vi "Test FlexiFlowInterfaceCH2 API.vi"() -> ()   [LabVIEW 2025]
doc: "FlexiFlowInterfaceCH2 API Tester."
uses:
  <vilib>/MGI/Panel Manager/Panel/Panel.lvlib
  <vilib>/MGI/Panel Manager/Panel/Panel/Window/Window.vi
  <vilib>/MGI/Panel Manager/Panel/Panel/Window/Window.lvclass
  <vilib>/MGI/Panel Manager/Panel/Panel/Subpanel/Subpanel.vi
  <vilib>/MGI/Panel Manager/Panel/Panel/Subpanel/Subpanel.lvclass
  <vilib>/MGI/Panel Manager/Panel/Panel/Window/Dialog/Dialog.vi
  <vilib>/MGI/Panel Manager/Panel/Panel/Window/Dialog/Dialog.lvclass
  C:/Program Files/National Instruments/LabVIEW 2025/vi.lib/MGI/Panel Manager/Panel/Panel/Panel.lvclass
  C:/Program Files/National Instruments/LabVIEW 2025/vi.lib/MGI/Panel Manager/Panel/Panel/Window/Window.lvclass
  C:/Program Files/National Instruments/LabVIEW 2025/vi.lib/MGI/Panel Manager/Panel/Panel/Window/Dialog/Dialog.lvclass
  C:/Program Files/National Instruments/LabVIEW 2025/vi.lib/MGI/Panel Manager/Panel/Panel/Subpanel/Subpanel.lvclass
  FlexiFlowInterface/Modbus TCP Connection Settings--cluster.ctl
  FlexiFlowInterface/FlexiFlowDevice--enum.ctl
  phlair-shared-libraries/Modbus Flexi-Flow API/Control Function Values--enum.ctl
  phlair-shared-libraries/Modbus Flexi-Flow API/Bronkhorst Flexi-Flow ModbusTCP API.lvlib
  FlexiFlowInterface/Modbus Flexi-Flow Controls--cluster.ctl
  FlexiFlowInterface/Modbus Flexi-Flow Measure State--cluster.ctl
  <vilib>/Plasmionique/MB Master/MB_Master_TCP/MB_Master_TCP.lvclass
  FlexiFlowInterface/Modbus Flexi-Flow State--cluster.ctl
  phlair-shared-libraries/Modbus Flexi-Flow API/Counter Setpoint Mode--enum.ctl
  phlair-shared-libraries/Modbus Flexi-Flow API/Counter Modes--enum.ctl
  FlexiFlowInterface/Counter Settings--cluster.ctl
  phlair-shared-libraries/Modbus Flexi-Flow API/Control Mode--enum.ctl
  phlair-shared-libraries/Modbus Flexi-Flow API/Capacity Units (Standard Volume Flow).ctl
  FlexiFlowInterface/Device Type--enum.ctl
panel:
  in  "Tab Control":T1(tab)
  out "Module Running?":bool
  in  "Show Module Panel":bool
  in  "Hide Module Panel":bool
  in  "Start Module":bool
  in  "Stop Module":bool
  in  "Show Block Diagram":bool
  in  "Tab Control":enum32{"Status", "Subpanel"}(tab)
  out "Status":string
  in  "Autoshow?":bool
  in  "Panel Type":enum16{"Window", "Dialog", "Subpanel"}(ring)
  in  "Change Panel":bool
  in  "Initialise Modbus Connections":bool
  in  "Wink Devices":bool
  in  "Flexi-Flow Conn":T2[](array[typedef])=[{"Label"="H2_PR", "Slave ID (255)"=255, "IP Address"="192.168.100.10", "Port (502)"=502, "Timeout (10000)"=2000}, {"Label"="N2_PR", "Slave ID (255)"=255, "IP Address"="192.168.100.20", "Port (502)"=502, "Timeout (10000)"=2000}, {"Label"="C_MFM", "Slave ID (255)"=255, "IP Address"="192.168.100.30", "Port (502)"=502, "Timeout (10000)"=2000}, {"Label"="A_MFC", "Slave ID (255)"=255, "IP Address"="192.168.100.40", "Port (502)"=502, "Timeout (10000)"=2000}]
  in  "Setpoint Slope":u16
  in  "Set Setpoint Slope":bool
  in  "Set Flow Capacity Unit":bool
  in  "Forwardpressure SP":dbl
  in  "Set Forward Pressure SP":bool
  in  "Backpressure SP":dbl
  in  "Set Backpressure Setpoint":bool
  in  "Flow SP":dbl
  in  "Set Flow SP":bool
  in  "Function":T3=enum."Downstream pressure"
  in  "Set Control Function":bool
  in  "Control Mode":T4 items=["Bus/RS232"=0, "FLOW-BUS slave"=2, "Valve close"=3, "Controller idle"=4, "Setpoint 100%"=7, "Valve fully open"=8, "Calibration mode"=9, "Setpoint 0%"=12, "RS232"=18, "Valve steering"=20, "Valve safe state"=22]
  in  "Set Control Mode":bool
  in  "User Tag":string
  in  "Set Device User Tag":bool
  in  "Device":T5
  in  "Standard Volume Flow":T6=4 items=["uls/h", "uls/min", "uls/s", "mls/h", "mls/min", "mls/s", "ls/h", "ls/min", "ls/s", "ccs/h", "ccn/min", "ccs/s", "mm3s/h", "mm3s/m", "mm3s/s", "cm3s/h", "cm3s/m", "cm3s/s", "m3s/h", "m3s/min", "m3s/s"]
  in  "Get Device Configuration":bool
  in  "Read Counter Unit":bool
  in  "Read Device User Tag":bool
  in  "Wink Device":bool
  in  "Read Fmeasure":bool
  out "Flexi-Flow Devices":T7[](array[typedef]) {"Control State"."Control Mode" items=["Bus/RS232"=0, "FLOW-BUS slave"=2, "Valve close"=3, "Controller idle"=4, "Setpoint 100%"=7, "Valve fully open"=8, "Calibration mode"=9, "Setpoint 0%"=12, "RS232"=18, "Valve steering"=20, "Valve safe state"=22]}
  in  "Device 2":T5 caption="Device"
  out "Data Table":map{string, dbl}(c390)
  in  "Counter Settings":T11={"Counter Setpoint Mode"=enum."No setpoint change (default)", "Counter Limit"=0.0, "Unit"="ls", "Counter Mode"=enum."Counter off (default)", "Counter New Setpoint"=0}
  in  "Reset All Device Counters":bool
  in  "Set Counter Settings":bool
  in  "Modbus TCP Connection":T2={"Label"="", "Slave ID (255)"=255, "IP Address"="192.168.100.10", "Port (502)"=502, "Timeout (10000)"=10000}
  in  "Set Modbus Configuration":bool
  # "This VI tests the API for the Module."
  # "Change Panel"
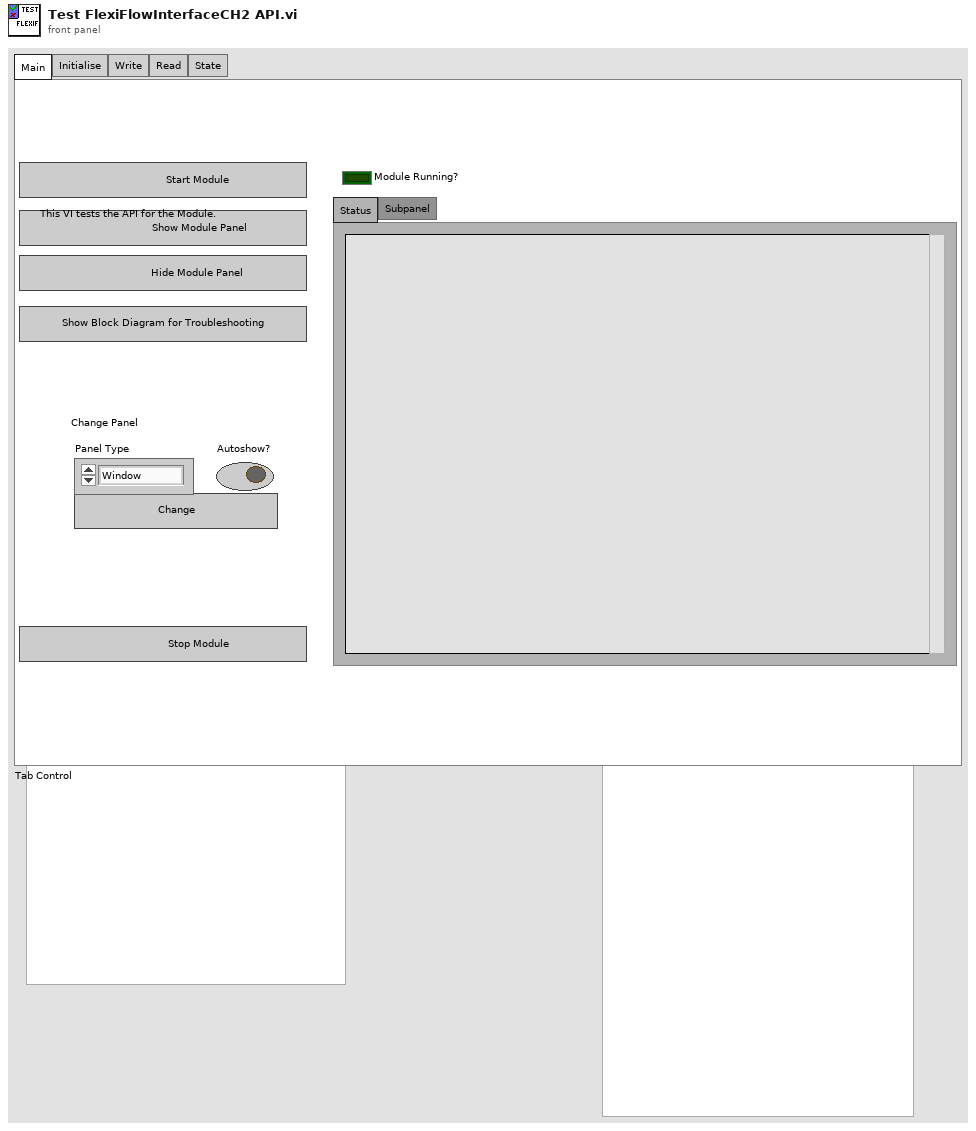
[diagram p1: front panel]
types:
  T1 = enum32{"Main", "Initialise", "Write", "Read", "State"}
  T2 = typedef "FlexiFlowInterface.lvlib/Modbus TCP Connection Settings--cluster.ctl" = cluster{"Label":string, "Slave ID (255)":u8, "IP Address":string, "Port (502)":u16, "Timeout (10000)":i32}
  T3 = typedef "Bronkhorst Flexi-Flow ModbusTCP API.lvlib/Control Function Values--enum.ctl" = enum16{"Flow", "Upstream pressure", "Downstream pressure", "Flow with upstream pressure limit", "Flow with downstream pressure limit", "Upstream pressure with flow limit", "Downstream pressure with flow limit"}
  T4 = typedef "Bronkhorst Flexi-Flow ModbusTCP API.lvlib/Control Mode--enum.ctl" = u16
  T5 = typedef "FlexiFlowInterface.lvlib/FlexiFlowDevice--enum.ctl" = enum16{"Hydrogen Inlet", "Nitrogen Inlet", "Cathode Outlet", "Anode Outlet"}
  T6 = typedef "Bronkhorst Flexi-Flow ModbusTCP API.lvlib/Capacity Units (Standard Volume Flow).ctl" = u16
  T7 = typedef "FlexiFlowInterface.lvlib/Modbus Flexi-Flow State--cluster.ctl" = cluster{"Type":T8, "Label":string, "User Tag":string, "MB_TCP session":refnum<class "MB_Master_TCP.lvclass">, "Control State":T9, "Measurement State":T10}
  T8 = typedef "FlexiFlowInterface.lvlib/Device Type--enum.ctl" = enum16{"Mass Flow Controller", "Mass Flow Meter"}
  T9 = typedef "FlexiFlowInterface.lvlib/Modbus Flexi-Flow Controls--cluster.ctl" = cluster{"Control Mode":T4, "Function":T3, "FSetpoint":sgl, "Flow Capacity Unit":string, "Setpoint Slope":u16, "P1Setpoint":sgl, "P2Setpoint":sgl}
  T10 = typedef "FlexiFlowInterface.lvlib/Modbus Flexi-Flow Measure State--cluster.ctl" = cluster{"Fmeasure":dbl, "P1measure":sgl, "P2measure":sgl}
  T11 = typedef "FlexiFlowInterface.lvlib/Counter Settings--cluster.ctl" = cluster{"Counter Setpoint Mode":T12, "Counter Limit":sgl, "Unit":string, "Counter Mode":T13, "Counter New Setpoint":u16}
  T12 = typedef "Bronkhorst Flexi-Flow ModbusTCP API.lvlib/Counter Setpoint Mode--enum.ctl" = enum16{"No setpoint change (default)", "Change setpoint to Counter new setpoint"}
  T13 = typedef "Bronkhorst Flexi-Flow ModbusTCP API.lvlib/Counter Modes--enum.ctl" = enum16{"Counter off (default)", "Counting up continuously", "Counting up until limit reached"}
  T14 = typedef "FlexiFlowInterface.lvlib/Broadcast Events--cluster.ctl" = cluster{"Module Did Init":refnum<user-event>, "Status Updated":refnum<user-event>, "Error Reported":refnum<user-event>, "Module Did Stop":refnum<user-event>, "Update Module Execution Status":refnum<user-event>, "Broadcast Device States":refnum<user-event>, "Broadcast State (Data Map)":refnum<user-event>}
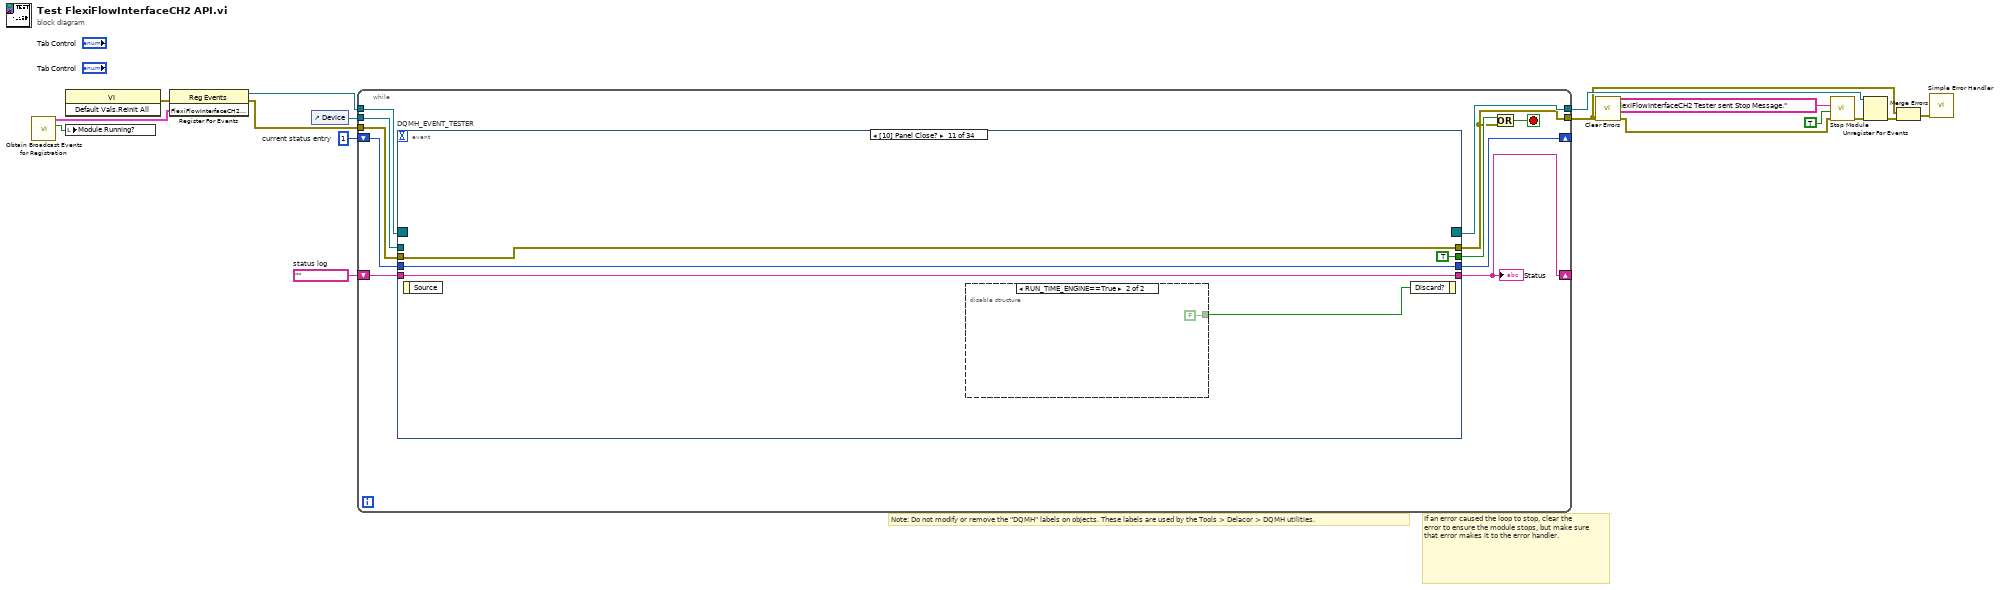
[diagram p0: block diagram]
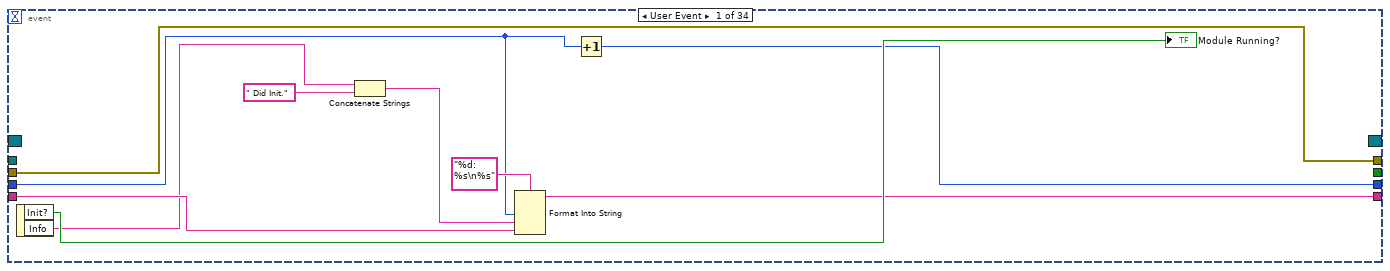
[diagram p2: hidden frame]
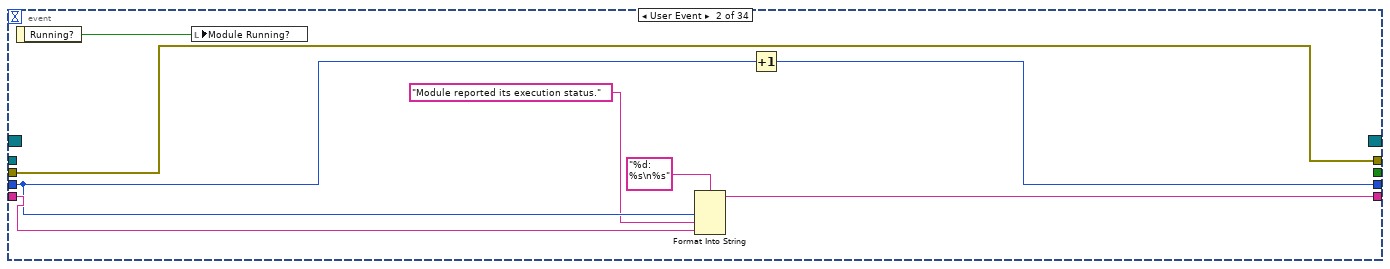
[diagram p3: hidden frame]
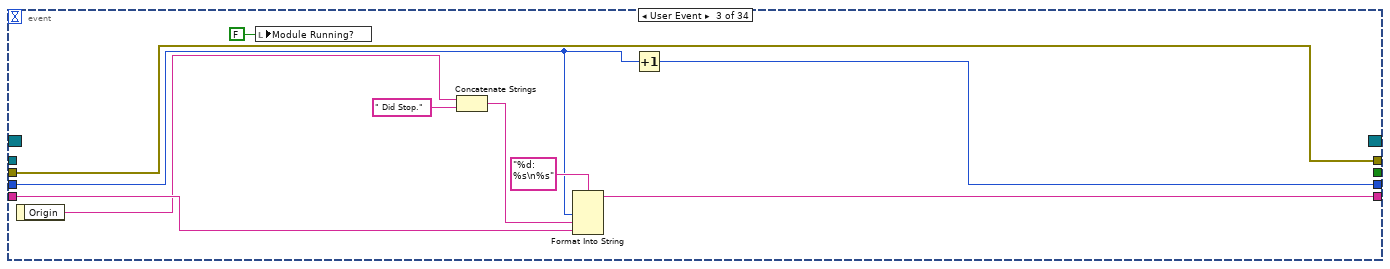
[diagram p4: hidden frame]
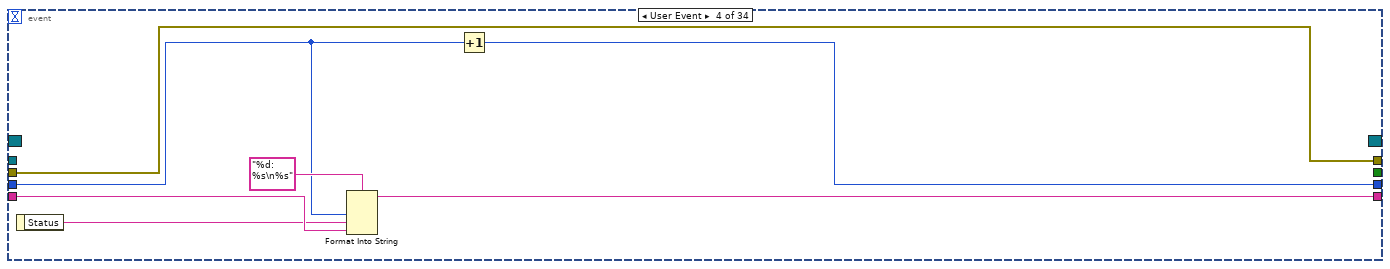
[diagram p5: hidden frame]
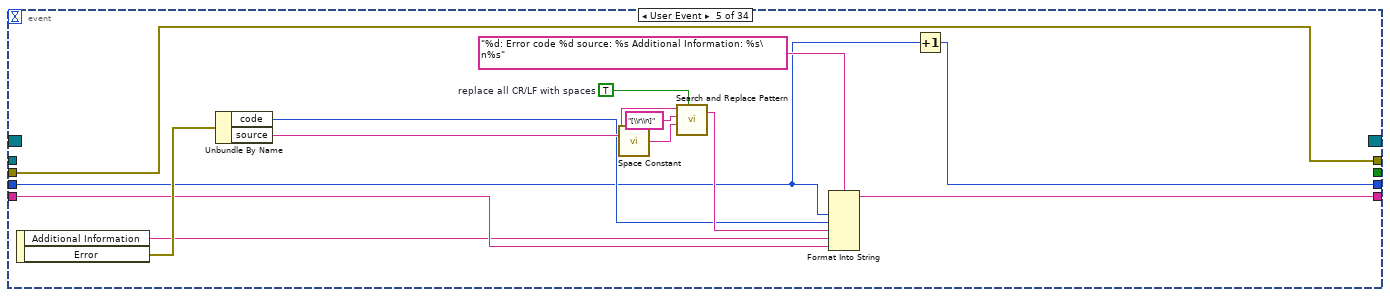
[diagram p6: hidden frame]
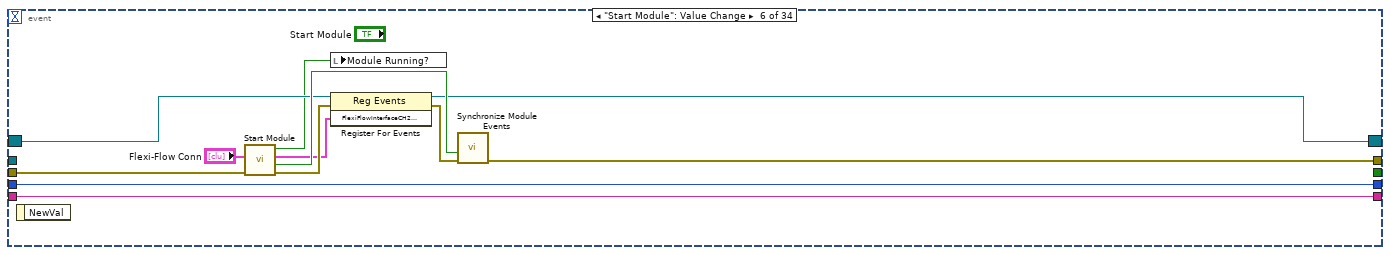
[diagram p7: hidden frame]
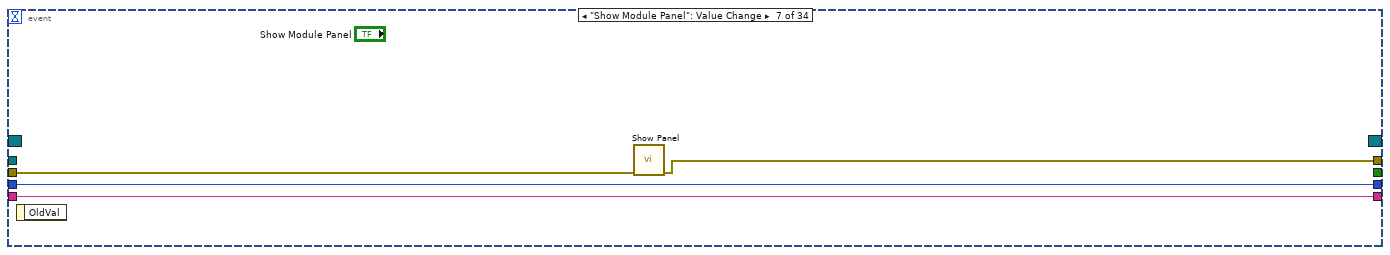
[diagram p8: hidden frame]
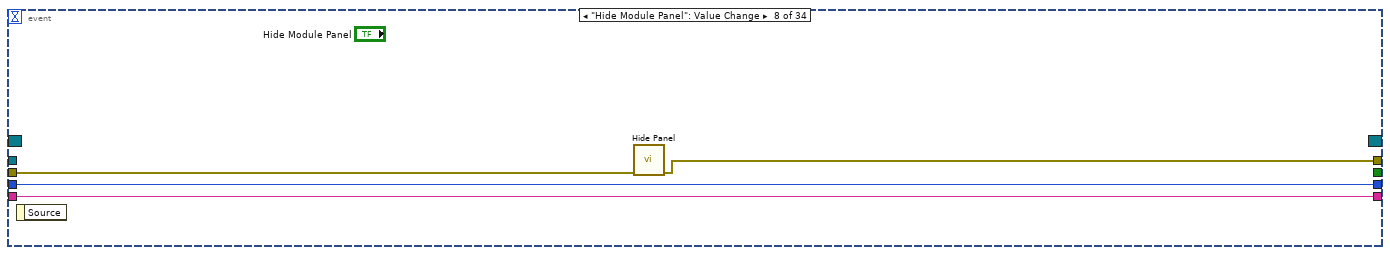
[diagram p9: hidden frame]
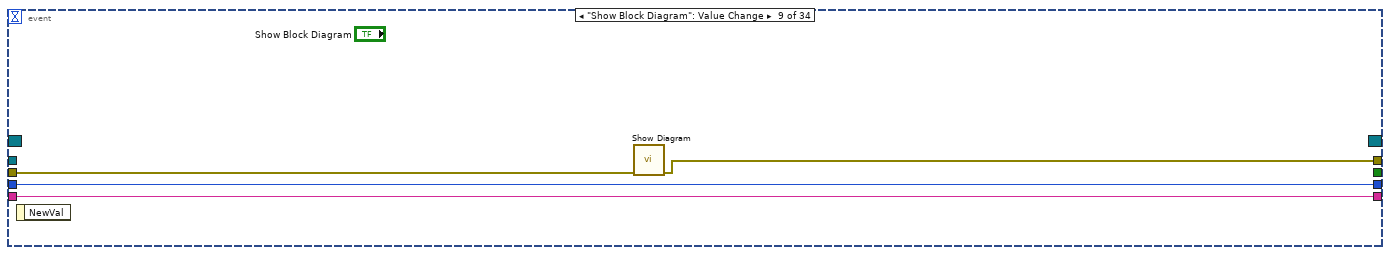
[diagram p10: hidden frame]
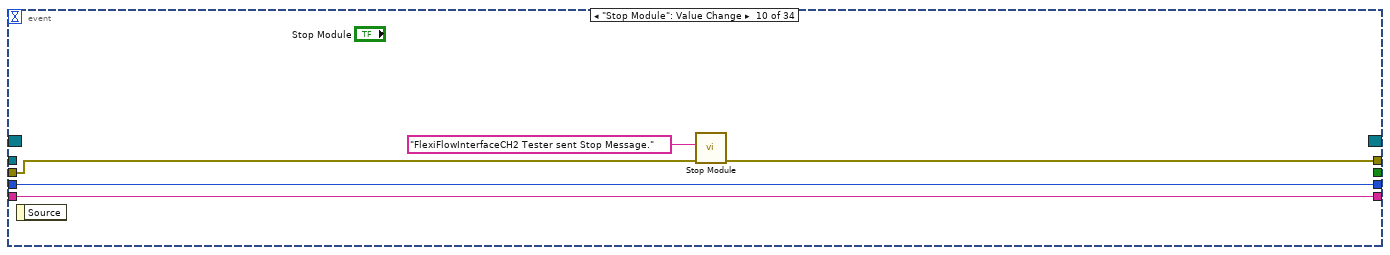
[diagram p11: hidden frame]
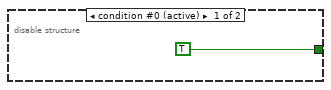
[diagram p12: hidden frame]
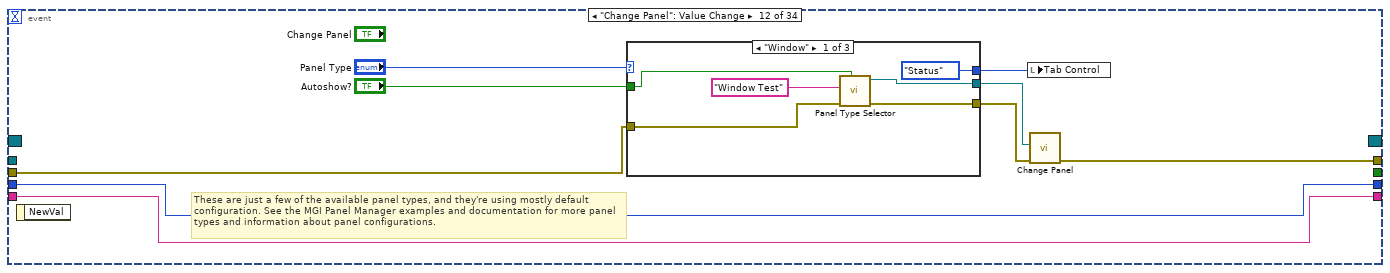
[diagram p13: hidden frame]
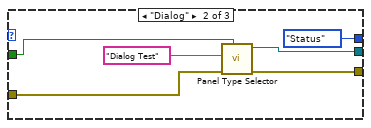
[diagram p14: hidden frame]
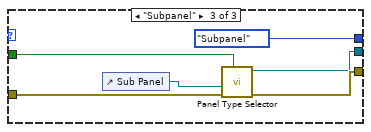
[diagram p15: hidden frame]
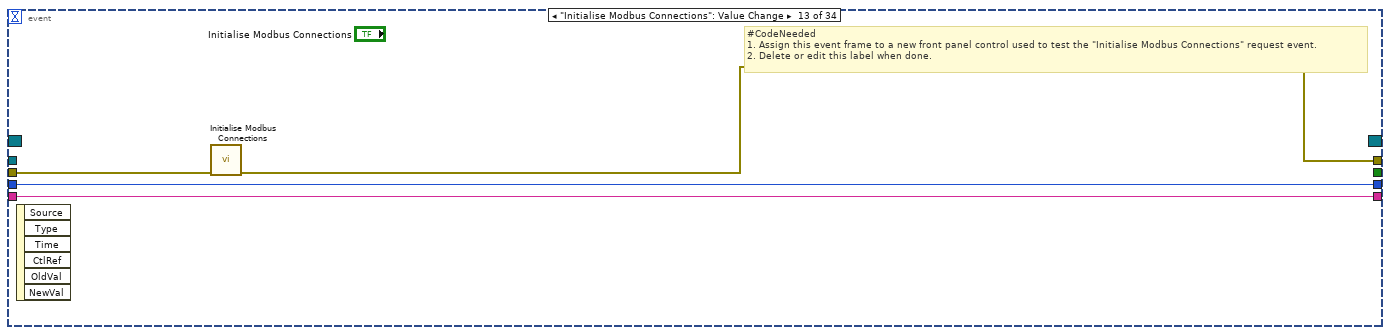
[diagram p16: hidden frame]
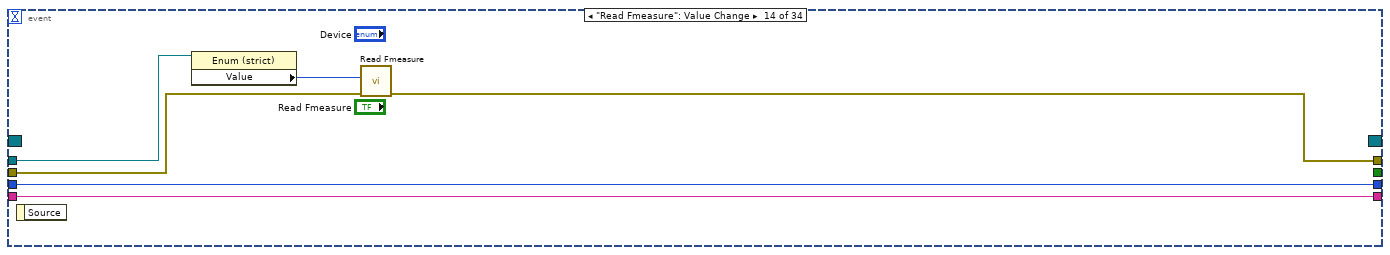
[diagram p17: hidden frame]
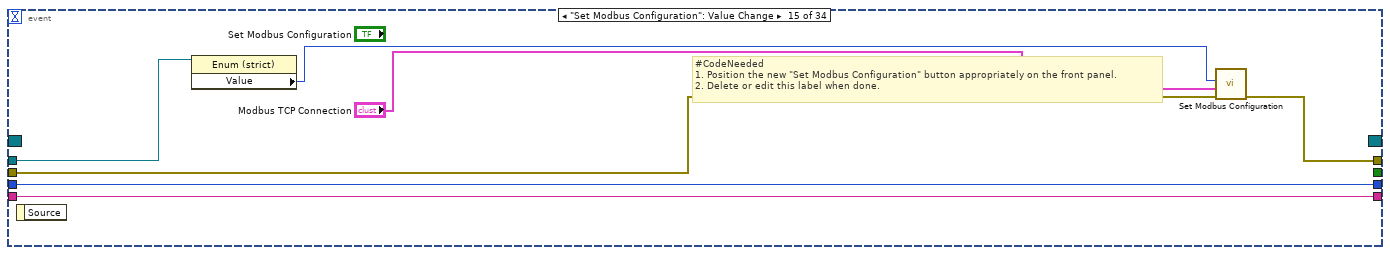
[diagram p18: hidden frame]
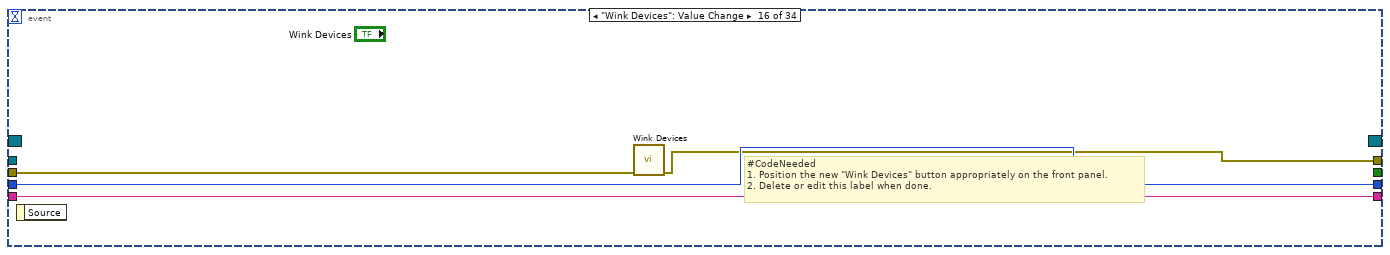
[diagram p19: hidden frame]
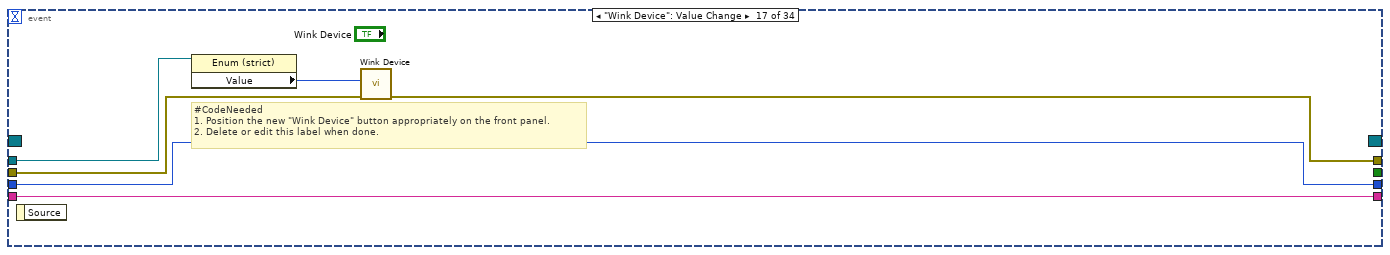
[diagram p20: hidden frame]
diagram:
  w12 = 1  # current status entry
  w13 = ""  # status log
  # "If an error caused the loop to stop, clear the error to ensure the module stops, but make sure that error makes it to the error handler."
  # "Note: Do not modify or remove the \"DQMH\" labels on objects. These labels are used by the Tools > Delacor > DQMH utilities."
  n1 = call "Obtain Broadcast Events for Registration.vi"() -> ("Already running?"=w2:bool, "FlexiFlowInterfaceCH2 Broadcast Events"=w9:T14)  [unwired: 9 in, 1 out]
  n2 = invoke class="VI" method="Default Vals.Reinit All"() -> (error out=w11:errorcluster)  [unwired: 3 in, 2 out]
  n3 = local write "Module Running?"(w2) -> ()
  n4 = register-events(error in=w11, w9) -> (reference out=w8:refnum<event-registration>, error out=w10:errorcluster)  [unwired: 1 in]
  n5 = control-ref of="Device"() -> (w1:refnum<vi>)
  n6 = while {
    tunnel: w8 -> [w27]
    tunnel: [w18] -> w3
    shift-right: [w22] -> _
    shift-left: w13 -> [w24]
    shift-right: [w23] -> _
    shift-left: w12 -> [w25]
    tunnel: w10 -> [w20]
    tunnel: [w19] -> w7
    tunnel: w1 -> [w17]
    stop <- w21 stop-if-true
    n7 = event "DQMH_EVENT_TESTER" shown="[10] Panel Close?" {
      selector: w27 -> [_ _ _ _ _ w82 _ _ _ _ _ _ _ _ _ _ _ _ _ _ _ _ _ _ _ _ _ _ _ _ _ _ _ _]
      dyn-events: [_ _ _ _ _ w81 _ _ _ _ _ _ _ _ _ _ _ _ _ _ _ _ _ _ _ _ _ _ _ _ _ _ _ _] -> w19
      timeout: _ -> [_ _ _ _ _ _ _ _ _ _ _ _ _ _ _ _ _ _ _ _ _ _ _ _ _ _ _ _ _ _ _ _ _ _]
      tunnel: [_ _ _ _ _ _ _ _ _ _ TRUE ("Discard?") _ _ _ _ _ _ _ _ _ _ _ _ _ _ _ _ _ _ _ _ _ _ _] -> w26
      tunnel: [w37 w39 w46 w56 w76 w80 w92 w96 w97 w103 w107 w119 w140 w146 w153 w157 w163 w170 w177 w184 w191 w198 w205 w218 w228 w232 w236 w242 w249 w255 w262 w268 w275 w279] -> w18
      tunnel: w25 -> [w33 w43 w53 w59 w66 w85 w90 w94 w98 w104 w108 w120 w141 w147 w154 w158 w164 w171 w178 w185 w192 w199 w206 w215 w225 w233 w237 w243 w250 w256 w263 w269 w273 w277]
      tunnel: w24 -> [w34 w44 w54 w58 w64 w86 w91 w95 w99 w105 w109 w121 w142 w148 w155 w159 w165 w172 w179 w186 w193 w200 w207 w217 w227 w234 w238 w244 w251 w257 w264 w270 w274 w278]
      tunnel: [w31 w41 w51 w60 w67 w86 w91 w95 w99 w105 w109 w121 w142 w148 w155 w159 w165 w172 w179 w186 w193 w200 w207 w216 w226 w234 w238 w244 w251 w257 w264 w270 w274 w278] -> w22
      tunnel: [w32 w42 w52 w62 w65 w85 w90 w94 w98 w104 w108 w120 w141 w147 w154 w158 w164 w171 w178 w185 w192 w199 w206 w214 w224 w233 w237 w243 w250 w256 w263 w269 w273 w277] -> w23
      tunnel: w20 -> [w37 w39 w46 w56 w76 w78 w89 w93 w100 w101 w107 w118 w143 w149 w156 w160 w166 w173 w180 w187 w194 w201 w208 w218 w228 w235 w239 w245 w252 w258 w265 w271 w275 w279]
      tunnel: w17 -> [_ _ _ _ _ _ _ _ _ _ _ _ _ w145 w152 _ w161 w168 w176 w182 w190 w197 w203 _ _ w231 _ w240 w248 w254 w261 w266 _ _]
      event User Event {
        n8 = event-data() -> ("Init?"=→"Module Running?":bool, "Info"=w30:string)  [unwired: 1 in]
        n9 = Concatenate Strings(w30, " Did Init.") -> (w29:string)
        n10 = Format Into String(format string="%d: %s\n%s", w33, w29, w34) -> (resulting string=w31:string)  [unwired: 2 in, 1 out]
        n11 = Increment(x=w33) -> (x+1=w32:i32)
      }
      event User Event {
        n12 = event-data() -> ("Running?"=w38:bool)  [unwired: 1 in]
        n13 = local write "Module Running?"(w38) -> ()
        n14 = Format Into String(format string="%d: %s\n%s", w43, "Module reported its execution status.", w44) -> (resulting string=w41:string)  [unwired: 2 in, 1 out]
        n15 = Increment(x=w43) -> (x+1=w42:i32)
      }
      event User Event {
        n16 = event-data() -> ("Origin"=w50:string)  [unwired: 1 in]
        n17 = local write "Module Running?"(FALSE ("Module Did Init?")) -> ()
        n18 = Concatenate Strings(w50, " Did Stop.") -> (w49:string)
        n19 = Format Into String(format string="%d: %s\n%s", w53, w49, w54) -> (resulting string=w51:string)  [unwired: 2 in, 1 out]
        n20 = Increment(x=w53) -> (x+1=w52:i32)
      }
      event User Event {
        n21 = event-data() -> ("Status"=w57:string)  [unwired: 1 in]
        n22 = Format Into String(format string="%d: %s\n%s", w59, w57, w58) -> (resulting string=w60:string)  [unwired: 2 in, 1 out]
        n23 = Increment(x=w59) -> (x+1=w62:i32)
      }
      event User Event {
        w72 = TRUE  # replace all CR/LF with spaces
        n24 = event-data() -> ("Additional Information"=w63:string, "Error"=w68:errorcluster)  [unwired: 1 in]
        n25 = Unbundle By Name(w68) -> ("code"=w69:i32, "source"=w70:string)
        n26 = call <vilib>:"Space Constant.vi"() -> ("String"=w73:string)
        n27 = call <vilib>:"Search and Replace Pattern.vi"("string"=w70, "regular expression (\"\")"="[\\r\\n]" ("regular expression (\"\")"), "replace string (\"\")"=w73, "replace all? (F)"=w72) -> ("result string"=w71:string)  [unwired: 1 in, 1 out]
        n28 = Format Into String(format string="%d: Error code %d source: %s Additional Information: %s\n%s", w66, w69, w71, w63, w64) -> (resulting string=w67:string)  [unwired: 2 in, 1 out]
        n29 = Increment(x=w66) -> (x+1=w65:i32)
      }
      event "Start Module": Value Change {
        n30 = event-data() -> ()  [unwired: 1 in, 1 out]
        n31 = call "Start Module.vi"("error in (no error)"=w78, "Flexi-Flow Conn"="Flexi-Flow Conn") -> ("error out"=w87:errorcluster, "Wait for Event Sync?"=w84:bool, "FlexiFlowInterfaceCH2 Broadcast Events"=w83:T14, "Module Was Already Running?"=w79:bool)  [unwired: 6 in]
        n32 = local write "Module Running?"(w79) -> ()
        n33 = register-events(reference=w82, error in=w87, w83) -> (reference out=w81:refnum<event-registration>, error out=w88:errorcluster)
        n34 = call "Synchronize Module Events.vi"("error in (no error)"=w88, "Wait for Event Sync?"=w84) -> ("error out"=w80:errorcluster)  [unwired: 9 in]
      }
      event "Show Module Panel": Value Change {
        n35 = event-data() -> ()  [unwired: 1 in, 1 out]
        n36 = call "Show Panel.vi"("error in (no error)"=w89) -> ("error out"=w92:errorcluster)  [unwired: 10 in]
      }
      event "Hide Module Panel": Value Change {
        n37 = event-data() -> ()  [unwired: 1 in, 1 out]
        n38 = call "Hide Panel.vi"("error in (no error)"=w93) -> ("error out"=w96:errorcluster)  [unwired: 10 in]
      }
      event "Show Block Diagram": Value Change {
        n39 = event-data() -> ()  [unwired: 1 in, 1 out]
        n40 = call "Show Diagram.vi"("error in (no error)"=w100) -> ("error out"=w97:errorcluster)  [unwired: 10 in]
      }
      event "Stop Module": Value Change {
        n41 = event-data() -> ()  [unwired: 1 in, 1 out]
        n42 = call "Stop Module.vi"("error in (no error)"=w101, "Origin"="FlexiFlowInterfaceCH2 Tester sent Stop Message.") -> ("error out"=w103:errorcluster)  [unwired: 9 in]
      }
      event Panel Close? {
        n43 = event-data() -> ()  [unwired: 1 in, 1 out]
        n44 = disable-structure shown="RUN_TIME_ENGINE==True" {
          disable-tunnel: [TRUE ("Discard?") FALSE ("Discard?")] -> w110
          frame condition #0 (active) {
          }
          frame condition #1 {
          }
        }
        n45 = event-data("Discard?"=w110) -> ()  [unwired: 1 in, 1 out]
      }
      event "Change Panel": Value Change {
        # "These are just a few of the available panel types, and they're using mostly default configuration. See the MGI Panel Manager examples and documentation for more panel types and information about panel configurations."
        n46 = event-data() -> ()  [unwired: 1 in, 1 out]
        n47 = case shown="\"Window\"" "Panel Type" {
          tunnel: w118 -> [w127 w133 w139]
          tunnel: [w126 w132 w138] -> w117
          tunnel: [w125 w131 w137] -> w116
          tunnel: [enum32{"Status", "Subpanel"}."Status" ("Tab Control") enum32{"Status", "Subpanel"}."Status" ("Tab Control") enum32{"Status", "Subpanel"}."Subpanel" ("Tab Control")] -> w114
          tunnel: "Autoshow?" -> [w122 w128 w134]
          frame "Window" {
            n48 = call-poly <vilib>:"Panel Type Selector.vi"("Autoshow? (T)"=w122, "error in (no error)"=w127, "Default Title"="Window Test") -> ("error out"=w126:errorcluster, "Window out"=w125:refnum<class "Window.lvclass">)  [unwired: 7 in]
          }
          frame "Dialog" {
            n49 = call-poly <vilib>:"Panel Type Selector.vi"("Autoshow? (T)"=w128, "Error In"=w133, "Default Title"="Dialog Test") -> ("Error Out"=w132:errorcluster, "Dialog out"=w131:refnum<class "Dialog.lvclass">)  [unwired: 7 in]
          }
          frame "Subpanel" {
            n50 = control-ref of="Sub Panel"() -> (w136:refnum<vi>)
            n51 = call-poly <vilib>:"Panel Type Selector.vi"("Autoshow? (T)"=w134, "Error In"=w139, "Sub Panel"=w136) -> ("Error Out"=w138:errorcluster, "Subpanel Out"=w137:refnum<class "Subpanel.lvclass">)  [unwired: 7 in]
          }
        }
        n52 = local write "Tab Control"(w114) -> ()
        n53 = call "Change Panel.vi"("error in (no error)"=w117, "New Panel"=w116) -> ("error out"=w119:errorcluster)  [unwired: 9 in]
      }
      event "Initialise Modbus Connections": Value Change {
        # "#CodeNeeded\n1. Assign this event frame to a new front panel control used to test the \"Initialise Modbus Connections\" request event.\n2. Delete or edit this label when done."
        n54 = event-data() -> ()  [unwired: 1 in, 6 out]
        n55 = call "Initialise Modbus Connections.vi"("error in"=w143) -> ("error out"=w140:errorcluster)  [unwired: 10 in]
      }
      event "Read Fmeasure": Value Change {
        n56 = event-data() -> ()  [unwired: 1 in, 1 out]
        n57 = property class="Enum (strict)"(reference=w145) -> ("Value"=w144:T5)  [unwired: 1 in, 2 out]
        n58 = call "Read Fmeasure.vi"("error in"=w149, "Device"=w144) -> ("error out"=w146:errorcluster)  [unwired: 9 in]
      }
      event "Set Modbus Configuration": Value Change {
        # "#CodeNeeded\n1. Position the new \"Set Modbus Configuration\" button appropriately on the front panel.\n2. Delete or edit this label when done."
        n59 = event-data() -> ()  [unwired: 1 in, 1 out]
        n60 = property class="Enum (strict)"(reference=w152) -> ("Value"=w150:T5)  [unwired: 1 in, 2 out]
        n61 = call "Set Modbus Configuration.vi"("error in"=w156, "Modbus TCP Connection"="Modbus TCP Connection", "Device"=w150) -> ("error out"=w153:errorcluster)  [unwired: 8 in]
      }
      event "Wink Devices": Value Change {
        # "#CodeNeeded\n1. Position the new \"Wink Devices\" button appropriately on the front panel.\n2. Delete or edit this label when done."
        n62 = event-data() -> ()  [unwired: 1 in, 1 out]
        n63 = call "Wink Devices.vi"("error in"=w160) -> ("error out"=w157:errorcluster)  [unwired: 10 in]
      }
      event "Wink Device": Value Change {
        # "#CodeNeeded\n1. Position the new \"Wink Device\" button appropriately on the front panel.\n2. Delete or edit this label when done."
        n64 = event-data() -> ()  [unwired: 1 in, 1 out]
        n65 = property class="Enum (strict)"(reference=w161) -> ("Value"=w162:T5)  [unwired: 1 in, 2 out]
        n66 = call "Wink Device.vi"("error in"=w166, "Device"=w162) -> ("error out"=w163:errorcluster)  [unwired: 9 in]
      }
      event "Set Control Function": Value Change {
        # "#CodeNeeded\n1. Position the new \"Set Control Function\" button appropriately on the front panel.\n2. Delete or edit this label when done."
        n67 = event-data() -> ()  [unwired: 1 in, 1 out]
        n68 = property class="Enum (strict)"(reference=w168) -> ("Value"=w169:T5)  [unwired: 1 in, 2 out]
        n69 = call "Set Control Function.vi"("error in"=w173, "Function"="Function", "Device"=w169) -> ("error out"=w170:errorcluster)  [unwired: 8 in]
      }
      event "Set Flow SP": Value Change {
        n70 = event-data() -> ()  [unwired: 1 in, 1 out]
        n71 = property class="Enum (strict)"(reference=w176) -> ("Value"=w175:T5)  [unwired: 1 in, 2 out]
        n72 = call "Set Flow Setpoint.vi"("error in"=w180, "Setpoint Value"="Flow SP", "Device"=w175) -> ("error out"=w177:errorcluster)  [unwired: 8 in]
      }
      event "Set Backpressure Setpoint": Value Change {
        n73 = event-data() -> ()  [unwired: 1 in, 1 out]
        n74 = property class="Enum (strict)"(reference=w182) -> ("Value"=w181:T5)  [unwired: 1 in, 2 out]
        n75 = call "Set Backpressure Setpoint.vi"("error in"=w187, "Backpressure SP"="Backpressure SP", "PDU Address 32-bit Float"=w181) -> ("error out"=w184:errorcluster)  [unwired: 8 in]
      }
      event "Set Forward Pressure SP": Value Change {
        # "#CodeNeeded\n1. Position the new \"Set Forward Pressure SP\" button appropriately on the front panel.\n2. Delete or edit this label when done."
        n76 = event-data() -> ()  [unwired: 1 in, 1 out]
        n77 = property class="Enum (strict)"(reference=w190) -> ("Value"=w189:T5)  [unwired: 1 in, 2 out]
        n78 = call "Set Forward Pressure SP.vi"("error in"=w194, "Pressure SP"="Forwardpressure SP", "Device"=w189) -> ("error out"=w191:errorcluster)  [unwired: 8 in]
      }
      event "Set Flow Capacity Unit": Value Change {
        # "#CodeNeeded\n1. Position the new \"Set Flow Capacity Unit\" button appropriately on the front panel.\n2. Delete or edit this label when done."
        n79 = event-data() -> ()  [unwired: 1 in, 1 out]
        n80 = property class="Enum (strict)"(reference=w197) -> ("Value"=w196:T5)  [unwired: 1 in, 2 out]
        n81 = call "Set Flow Capacity Unit.vi"("error in"=w201, "Standard Volume Flow"="Standard Volume Flow", "Device"=w196) -> ("error out"=w198:errorcluster)  [unwired: 8 in]
      }
      event "Set Setpoint Slope": Value Change {
        n82 = event-data() -> ()  [unwired: 1 in, 1 out]
        n83 = property class="Enum (strict)"(reference=w203) -> ("Value"=w202:T5)  [unwired: 1 in, 2 out]
        n84 = call "Set Setpoint Slope.vi"("error in"=w208, "Setpoint Slope"="Setpoint Slope", "Device"=w202) -> ("error out"=w205:errorcluster)  [unwired: 8 in]
      }
      event User Event {
        # "#CodeNeeded Replace this format string with a meaningful value for this broadcast, then wire broadcast data from the Event Data Node to the input(s) of the Format Into String function."
        # "#CodeNeeded\n1. Process the event data sent by the \"Broadcast Device States\" broadcast event.\n2. Delete or edit this label when done."
        n85 = event-data() -> ("Flexi-Flow Devices"=→"Flexi-Flow Devices":T7[])  [unwired: 1 in, 4 out]
        n86 = Format Into String(format string="Response Received - %s", "Device States" ("input 1")) -> (resulting string=w211:string)  [unwired: 2 in, 1 out]
        n87 = Increment(x=w215) -> (x+1=w214:i32)
        n88 = Format Into String(format string="%d: %s\n%s", w215, w211, w217) -> (resulting string=w216:string)  [unwired: 2 in, 1 out]
      }
      event User Event {
        # "#CodeNeeded Replace this format string with a meaningful value for this broadcast, then wire broadcast data from the Event Data Node to the input(s) of the Format Into String function."
        # "#CodeNeeded\n1. Process the event data sent by the \"Broadcast State (Data Map)\" broadcast event.\n2. Delete or edit this label when done."
        n89 = event-data() -> ("Data Table"=→"Data Table":map{string, dbl})  [unwired: 1 in, 4 out]
        n90 = Format Into String(format string="Response Received - %s", "Data Table" ("input 1")) -> (resulting string=w221:string)  [unwired: 2 in, 1 out]
        n91 = Increment(x=w225) -> (x+1=w224:i32)
        n92 = Format Into String(format string="%d: %s\n%s", w225, w221, w227) -> (resulting string=w226:string)  [unwired: 2 in, 1 out]
      }
      event "Set Counter Settings": Value Change {
        n93 = event-data() -> ()  [unwired: 1 in, 1 out]
        n94 = property class="Enum (strict)"(reference=w231) -> ("Value"=w230:T5)  [unwired: 1 in, 2 out]
        n95 = call "Set Counter Settings.vi"("error in"=w235, "Counter Settings"="Counter Settings", "Device"=w230) -> ("error out"=w232:errorcluster)  [unwired: 8 in]
      }
      event "Reset All Device Counters": Value Change {
        # "#CodeNeeded\n1. Position the new \"Reset All Device Counters\" button appropriately on the front panel.\n2. Delete or edit this label when done."
        n96 = event-data() -> ()  [unwired: 1 in, 1 out]
        n97 = call "Reset All Device Counters.vi"("error in"=w239) -> ("error out"=w236:errorcluster)  [unwired: 10 in]
      }
      event "Read Device User Tag": Value Change {
        # "#CodeNeeded\n1. Position the new \"Read Device User Tag\" button appropriately on the front panel.\n2. Delete or edit this label when done."
        n98 = event-data() -> ()  [unwired: 1 in, 1 out]
        n99 = property class="Enum (strict)"(reference=w240) -> ("Value"=w241:T5)  [unwired: 1 in, 2 out]
        n100 = call "Read Device User Tag.vi"("error in"=w245, "Device"=w241) -> ("error out"=w242:errorcluster)  [unwired: 9 in]
      }
      event "Set Device User Tag": Value Change {
        # "#CodeNeeded\n1. Position the new \"Set Device User Tag\" button appropriately on the front panel.\n2. Delete or edit this label when done."
        n101 = event-data() -> ()  [unwired: 1 in, 1 out]
        n102 = property class="Enum (strict)"(reference=w248) -> ("Value"=w247:T5)  [unwired: 1 in, 2 out]
        n103 = call "Set Device User Tag.vi"("error in"=w252, "User Tag"="User Tag", "Device"=w247) -> ("error out"=w249:errorcluster)  [unwired: 8 in]
      }
      event "Read Counter Unit": Value Change {
        # "#CodeNeeded\n1. Position the new \"Read Counter Unit\" button appropriately on the front panel.\n2. Delete or edit this label when done."
        n104 = event-data() -> ()  [unwired: 1 in, 1 out]
        n105 = property class="Enum (strict)"(reference=w254) -> ("Value"=w253:T5)  [unwired: 1 in, 2 out]
        n106 = call "Read Counter Unit.vi"("error in"=w258, "Device"=w253) -> ("error out"=w255:errorcluster)  [unwired: 9 in]
      }
      event "Set Control Mode": Value Change {
        # "#CodeNeeded\n1. Position the new \"Set Control Mode\" button appropriately on the front panel.\n2. Delete or edit this label when done."
        n107 = event-data() -> ()  [unwired: 1 in, 1 out]
        n108 = property class="Enum (strict)"(reference=w261) -> ("Value"=w260:T5)  [unwired: 1 in, 2 out]
        n109 = call "Set Control Mode.vi"("error in"=w265, "Control Mode"="Control Mode", "Device"=w260) -> ("error out"=w262:errorcluster)  [unwired: 8 in]
      }
      event "Get Device Configuration": Value Change {
        # "#CodeNeeded\n1. Position the new \"Get Device Configuration\" button appropriately on the front panel.\n2. Delete or edit this label when done."
        n110 = event-data() -> ()  [unwired: 1 in, 1 out]
        n111 = property class="Enum (strict)"(reference=w266) -> ("Value"=w267:T5)  [unwired: 1 in, 2 out]
        n112 = call "Get Device Configuration.vi"("error in"=w271, "Device"=w267) -> ("error out"=w268:errorcluster)  [unwired: 9 in]
      }
      event Value Change {
        n113 = event-data() -> ("NewVal"=w272:T5)  [unwired: 1 in, 5 out]
        n114 = local write "Device 2"(w272) -> ()
      }
      event Value Change {
        n115 = event-data() -> ("NewVal"=w276:T5)  [unwired: 1 in, 5 out]
        n116 = local write "Device"(w276) -> ()
      }
    }
    "Status" <- w22
    n117 = Or(x=w26, y=w18) -> (x .or. y?=w21:bool)
  }
  n118 = call <vilib>:"Clear Errors.vi"("error in (no error)"=w3) -> ("error out"=w5:errorcluster)  [unwired: 5 in, 1 out]
  n119 = call "Stop Module.vi"("error in (no error)"=w5, "Wait for Module to Stop? (F)"=TRUE ("Wait for Module to stop?"), "Origin"="FlexiFlowInterfaceCH2 Tester sent Stop Message.") -> ("error out"=w15:errorcluster)  [unwired: 8 in]
  n120 = Unregister For Events(event registration refnum=w7, error in=w15) -> (error out=w16:errorcluster)
  n121 = Merge Errors(w3, w16) -> (w4:errorcluster)
  n122 = call <vilib>:"Simple Error Handler.vi"("error in (no error)"=w4) -> ()  [unwired: 4 in, 5 out]
